vi "Triangle Window (CDB).vi"(0 "X":cdb[](array[numeric])) -> (1 "Windowed X":cdb[](array[numeric]), 2 "error":i32)   [LabVIEW 2014, in "NI_AALPro.lvlib"]
doc: "Applies a triangular window (Bartlett Window) to the input signal <B>X</B>. Wire data to the <B>X</B> input to determine the polymorphic instance to use or manually select the instance."
uses:
  NI_AALPro.lvlib
  lvanlys.dll
panel:
  # "Triangle Window"
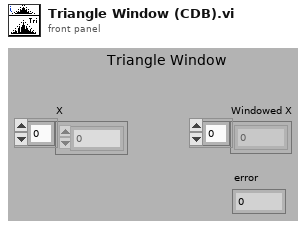
[diagram p1: front panel]
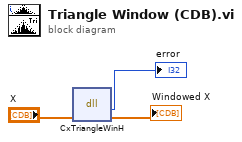
[diagram p0: block diagram]
diagram:
  n1 = dll-call lib="C:/Program Files (x86)/National Instruments/LabVIEW 2014/resource/lvanlys.*" fn="CxTriangleWinH"("X"="X") -> (→"error":i32, "X"=→"Windowed X":cdb[])  [unwired: 3 in, 2 out]
